vi "BCC_TEST.vi"() -> ()   [LabVIEW 2014]
panel:
  out "size(s) 2":i32
  out "output bit stream 3":i8[](array[numeric]) caption="output bit stream"
  out "size(s)":i32
  out "sum":i16
  out "error out":errorcluster
  out "Waveform Graph":i16[][](graph)
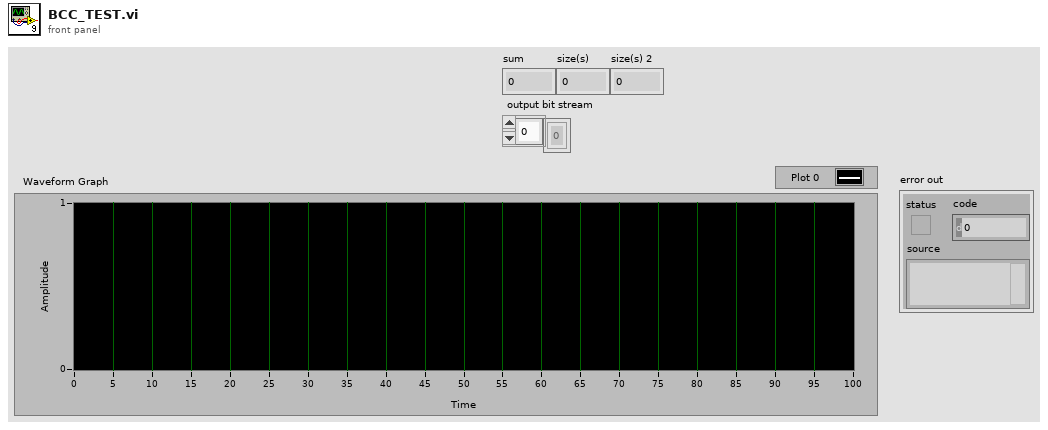
[diagram p1: front panel]
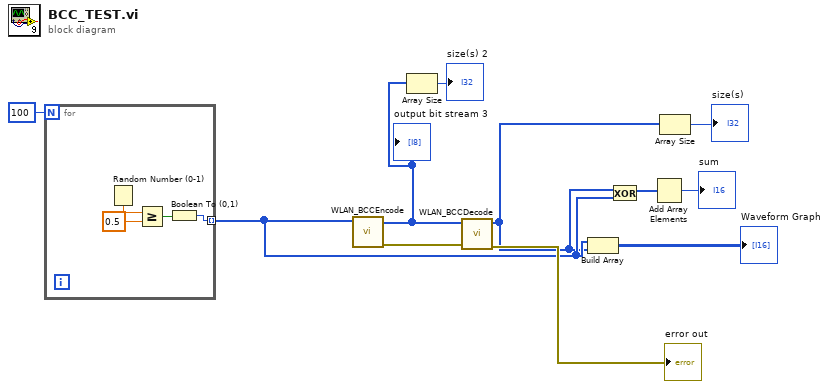
[diagram p0: block diagram]
diagram:
  n1 = for {
    N: 100 -> [_]
    tunnel: [w12] -> w7 mode=indexing
    n2 = Random Number (0-1)() -> (number: 0 to 1=w15:dbl)
    n3 = Greater Or Equal?(x=w15, y=0.5) -> (x >= y?=w13:bool)
    n4 = Boolean To (0,1)(Boolean=w13) -> (0, 1=w12:i16)
  }
  n5 = call "WLAN_BCCEncode.vi"("input bit stream"=w7) -> ("error out"=w9:errorcluster, "output bit stream 3"=w2:i8[])  [unwired: 9 in]
  "output bit stream 3" <- w2
  n6 = Array Size(array=w2) -> (size(s)=→"size(s) 2":i32)
  n7 = call "WLAN_BCCDecode.vi"("error in (no error)"=w9, "input bit stream"=w2) -> ("error out"=→"error out":errorcluster, "output bit stream"=w3:i8[])  [unwired: 8 in]
  n8 = Build Array(w7, w3) -> (→"Waveform Graph":i16[][])
  n9 = Exclusive Or(1:w7, 2:w3) -> (0:w5:i16[])
  n10 = Add Array Elements(numeric array=w5) -> (sum=→"sum":i16)
  n11 = Array Size(array=w3) -> (size(s)=→"size(s)":i32)
